vi "STOP_buttonGame.vi"() -> ()   [LabVIEW 2025]
uses:
  <vilib>/numeric/Random Number (Range) I64.vi
  <vilib>/numeric/sub_Random U32.vi
panel:
  in  "stop":bool
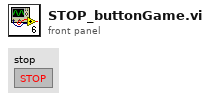
[diagram p1: front panel]
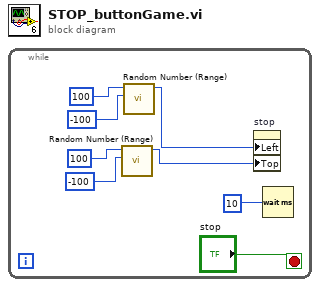
[diagram p0: block diagram]
diagram:
  n1 = while {
    stop <- "stop" stop-if-true
    n2 = call-poly <vilib>:"Random Number (Range).vi"("lower bound (-100)"=-100, "upper bound (100)"=100) -> ("number"=w1:i64)  [unwired: 9 in]
    n3 = call-poly <vilib>:"Random Number (Range).vi"("lower bound (-100)"=-100, "upper bound (100)"=100) -> ("number"=w5:i64)  [unwired: 9 in]
    n4 = property on="stop" class="Bool"("Left"=w5, "Top"=w1) -> ()  [unwired: 2 in, 2 out]
    n5 = Wait (ms)(milliseconds to wait=10) -> ()  [unwired: 1 out]
  }
